vi "Waveform Unflatten.vi"(7 "Header in":T1, 8 "error in (no error)":errorcluster, 10 "Data in in":T2[](array[typedef]), 11 "Flatten Data in":u8[](array[numeric])) -> (0 "error out":errorcluster, 2 "Data out":T2[](array[typedef]), 3 "Flatten Data out":u8[](array[numeric]), 5 "Header out":T1)   [LabVIEW 2021, in "CIFfifo.lvclass"]
uses:
  CIFfifo.lvclass
  typedef/Datatype Waveform.ctl
  typedef/FIFO Header.ctl
  CIFfifo.lvclass/CIFfifo.ctl
  ChannelCommon.lvlib
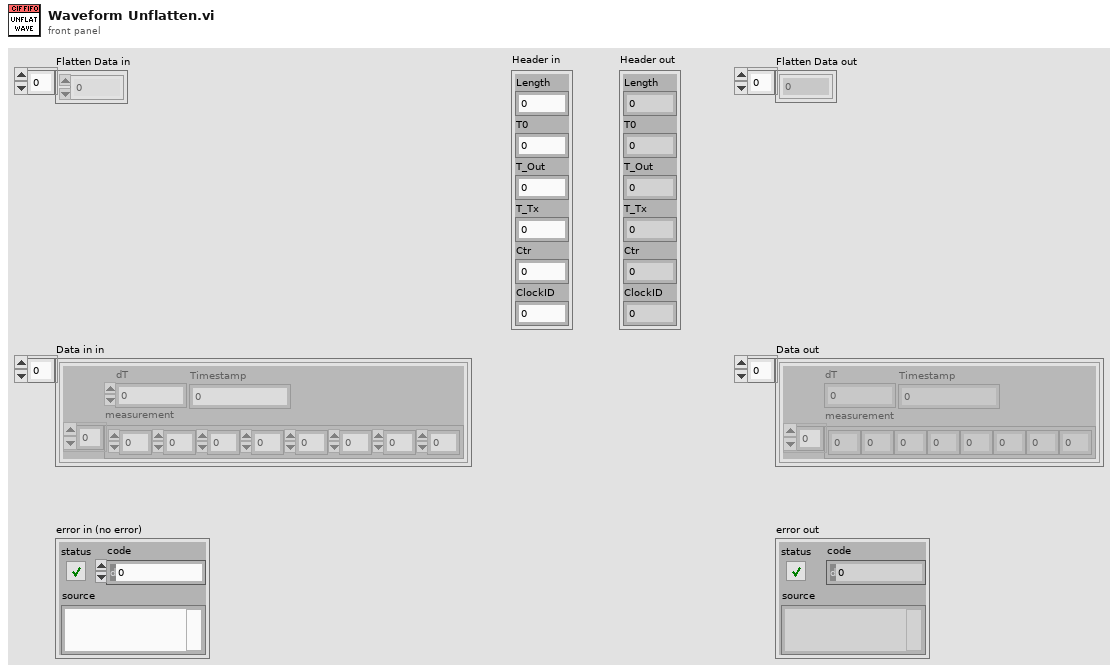
[diagram p1: front panel]
types:
  T1 = typedef "ChannelCommon.lvlib/FIFO Header.ctl" = cluster{"Length":u64, "T0":u64, "T_Out":u64, "T_Tx":u64, "Ctr":u64, "ClockID":u8}
  T2 = typedef "ChannelCommon.lvlib/Datatype Waveform.ctl" = cluster{"measurement":dbl[], "dT":dbl, "Timestamp":u64}
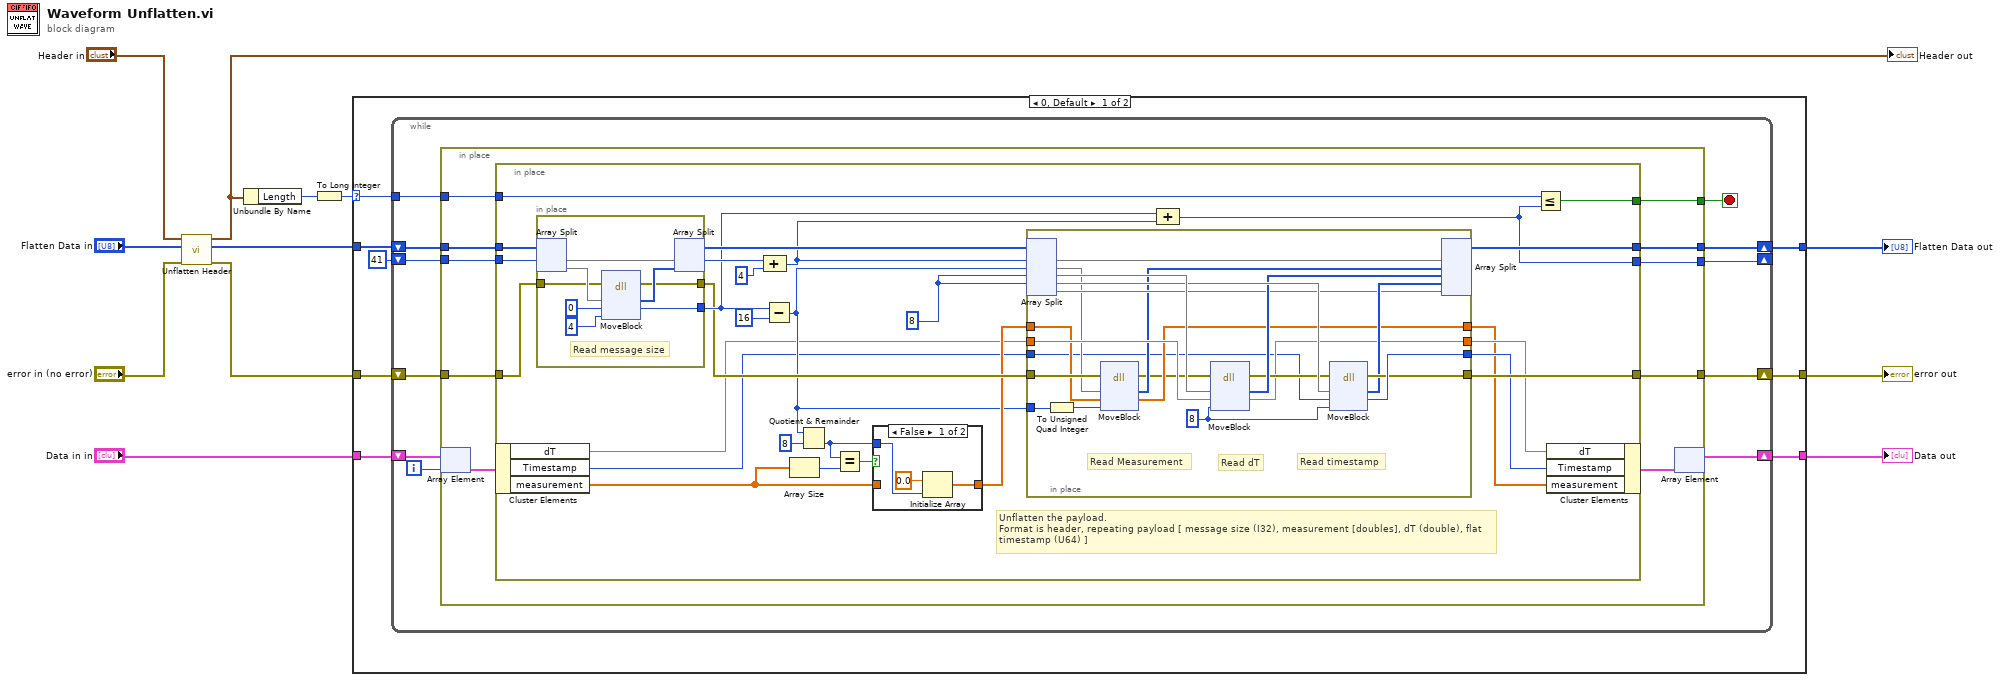
[diagram p0: block diagram]
diagram:
  n1 = call "Unflatten Header.vi"("error in"="error in (no error)", "Flattened Data in"="Flatten Data in", "Header in"="Header in") -> ("error out"=w6:errorcluster, "Flatten Data out"=w8:u8[], "Header out"=w3:T1)  [unwired: 6 in]
  "Header out" <- w3
  n2 = Unbundle By Name(w3) -> ("Length"=w4:u64)
  n3 = To Long Integer(number=w4) -> (32bit integer=w2:i32)
  n4 = case shown="0, Default" w2 {
    selector: w2 -> [w13 _]
    tunnel: [w20 w103] -> w12
    tunnel: "Data in in" -> [w19 w103]
    tunnel: [w17 w104] -> w10
    tunnel: [w16 w105] -> w9
    tunnel: w8 -> [w15 w105]
    tunnel: w6 -> [w14 w104]
    frame 0, Default {
      n5 = while {
        shift-right: [w27] -> w17
        shift-left: w14 -> [w28]
        shift-right: [w31] -> w16
        shift-left: w15 -> [w30]
        shift-right: [w25] -> _
        shift-left: 41 -> [w29]
        tunnel: w13 -> [w26]
        shift-right: [w21] -> w20
        shift-left: w19 -> [w23]
        i -> [w24]
        stop <- w22 stop-if-true
        n6 = in-place {
          in-place-border: [w41] -> w31
          in-place-border: w30 -> [w40]
          in-place-border: w29 -> [w39]
          in-place-border: w28 -> [w38]
          in-place-border: [w37] -> w27
          in-place-border: w26 -> [w36]
          in-place-border: [w35] -> w25
          in-place-border: [w34] -> w22
          n7 = in-place-array #1(w23, w24) -> (w33:T2)
          n8 = in-place {
            in-place-border: [w69] -> w41
            in-place-border: w40 -> [w68]
            in-place-border: w39 -> [w67]
            in-place-border: w38 -> [w66]
            in-place-border: [w65] -> w37
            in-place-border: w36 -> [w64]
            in-place-border: [w63] -> w35
            in-place-border: [w48] -> w34
            w52 = 8
            # "Unflatten the payload.\nFormat is header, repeating payload [ message size (I32), measurement [doubles], dT (double), flat timestamp (U64) ]"
            n9 = in-place-cluster #2(w33) -> ("dT"=w47:dbl, "Timestamp"=w46:u64, "measurement"=w43:dbl[])
            n10 = in-place {
              in-place-border: w66 -> [w79]
              in-place-border: [w75] -> w57
              in-place-border: [w74] -> w56
              # "Read message size"
              n11 = in-place-split #3(w68, w67) -> (w81:u8[], w80:u8[])
              n12 = dll-call lib="LabVIEW" fn="MoveBlock"(error in=w79, "source"=w80, "dest"=0, "size"=u64 4) -> (error out=w74:errorcluster, "source"=w76:u8[], "dest"=w75:i32)  [unwired: 4 in, 1 out]
              n13 = in-place-split #3(w81, w76) -> (w61:u8[], w62:i32)
            }
            n14 = Compound Arithmetic op=ADD(w62, 4 ("value")) -> (w58:i32)
            n15 = Subtract(x=w57, y=16) -> (x-y=w51:i32)
            n16 = Array Size(array=w43) -> (size(s)=w55:i32)
            n17 = Quotient & Remainder(x=w51, y=8) -> (floor(x/y)=w50:i32)  [unwired: 1 out]
            n18 = Equal?(x=w50, y=w55) -> (x = y?=w54:bool)
            n19 = case shown="False" w54 {
              tunnel: w43 -> [_ w73]
              tunnel: [w70 w73] -> w53
              tunnel: w50 -> [w72 _]
              frame False {
                n20 = Initialize Array(0.0, w72) -> (w70:dbl[])
              }
              frame True {
              }
            }
            n21 = in-place {
              in-place-border: [w86] -> w42
              in-place-border: [w91] -> w45
              in-place-border: [w100] -> w65
              in-place-border: w56 -> [w90]
              in-place-border: [w101] -> w44
              in-place-border: w53 -> [w87]
              in-place-border: w51 -> [w99]
              in-place-border: w47 -> [w97]
              in-place-border: w46 -> [w82]
              w83 = u64 8 ("size")
              # "Read timestamp"
              # "Read dT"
              # "Read Measurement"
              n22 = in-place-split #4(w61, w58, w51, w52, w52) -> (w102:u8[], w89:u8[], w98:u8[], w96:u8[], w92:u8[])
              n23 = To Unsigned Quad Integer(1:w99) -> (0:w84:u64)
              n24 = dll-call lib="LabVIEW" fn="MoveBlock"(error in=w90, "source"=w89, "dest"=w87, "size"=w84) -> (error out=w85:errorcluster, "source"=w88:u8[], "dest"=w86:dbl[])  [unwired: 4 in, 1 out]
              n25 = dll-call lib="LabVIEW" fn="MoveBlock"(error in=w85, "source"=w98, "dest"=w97, "size"=w83) -> (error out=w94:errorcluster, "source"=w95:u8[], "dest"=w91:dbl)  [unwired: 4 in, 1 out]
              n26 = dll-call lib="LabVIEW" fn="MoveBlock"(error in=w94, "source"=w96, "dest"=w82, "size"=w83) -> (error out=w100:errorcluster, "source"=w93:u8[], "dest"=w101:u64)  [unwired: 4 in, 1 out]
              n27 = in-place-split #4(w102, w88, w95, w93, w92) -> (w69:u8[])  [unwired: 4 out]
            }
            n28 = Compound Arithmetic op=ADD(w57, w58) -> (w63:i32)
            n29 = Less Or Equal?(x=w64, y=w63) -> (x <= y?=w48:bool)
            n30 = in-place-cluster #2("dT"=w45, "Timestamp"=w44, "measurement"=w42) -> (w32:T2)
          }
          n31 = in-place-array #1(w32) -> (w21:T2[])  [unwired: 1 out]
        }
      }
    }
    frame 40 {
      # "Header only"
    }
  }
  "Data out" <- w12
  "error out" <- w10
  "Flatten Data out" <- w9
